vi "Remaining_ms.vi"(7 "Time period target":i32 caption="Time period target [ms]", 11 "Error in":errorcluster caption="Error in (no error)", 12 "Start time in":i64=-1 caption="Start time in (-1: init) [ms]" min=-1 max=4294967295) -> (8 "Remaining time":i32 caption="Remaining time [ms]", 10 "Elapsed time":i32 caption="Elapsed time [ms]", 13 "Now":i64 caption="Now [ms]", 14 "Start time out":i64 caption="Start time out [ms]", 15 "Error out":errorcluster)   [LabVIEW 2017, in "GPTiming.lvlib"]
doc: "Calculates <B>Remaining time</B> of <B>Time period target</B> since <B>Start time in</B>.\n\n<B>Start time in</B> will be returned in <B>Start time out</B>. Set <B>Start time in</B> to -1 (or leave it unwired) to get the current time returned in <B>Start time out</B> instead. <B>Now</B> will always be the current time.\n\nThis VI uses the ms tick counter and will be able to count for 2^31-1 ms (almost 25 days) before <B>Remaining time</B> wraps around. <B>Remaining time</B> will be latched at 0 from when the remaining time runs out and until the tick counter wraps around. <B>Elapsed time</B> will continue counting up past the remaining time running out, thus you can use this output to see how late you were if you overshoot the <B>Time period target</B>.\n\nThis VI is inlined. <B>Error in</B> is wired straight through to <B>Error out</B> to enable optional dataflow dependency (offering control of when <B>Now</B> is).\n\nSteen Schmidt\nGPower\n6/12 2013"
uses:
  GPTiming.lvlib
panel:
  # "Copyright © 2013\nGPower\nSee enclosed license file for terms and conditions"
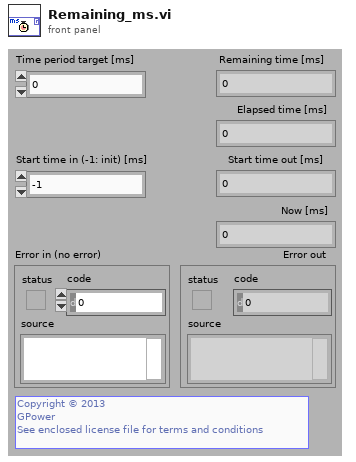
[diagram p1: front panel]
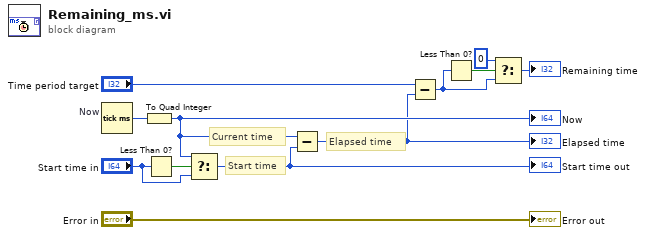
[diagram p0: block diagram]
diagram:
  # "Elapsed time"
  # "Current time"
  # "Start time"
  n1 = Tick Count (ms) "Now"() -> (millisecond timer value=w10:u32)
  n2 = To Quad Integer(1:w10) -> (0:w7:i64)
  "Now" <- w7
  n3 = Less Than 0?(x="Start time in") -> (x < 0?=w11:bool)
  n4 = Select(t=w7, s=w11, f="Start time in") -> (s? t:f=w8:i64)
  "Start time out" <- w8
  n5 = Subtract(x=w7, y=w8) -> (x-y=w1:i64)
  "Elapsed time" <- w1
  n6 = Subtract(x="Time period target", y=w1) -> (x-y=w3:i64)
  n7 = Less Than 0?(x=w3) -> (x < 0?=w4:bool)
  n8 = Select(t=i64 0, s=w4, f=w3) -> (s? t:f=→"Remaining time":i64)
  "Error out" <- "Error in"
